vi "Delete_Overlay_2Images-2.vi"(0 "Delete \nOverlay?":bool, 1 "1st Image IN":T1, 2 "2nd Image IN":T1, 3 "error IN":errorcluster, 4 "Stored Overlay":T1) -> (5 "1st Image OUT":T1, 6 "2nd Image OUT":T1, 7 "error OUT":errorcluster)   [LabVIEW 2013]
uses:
  <vilib>/vision/Image Controls.llb/IMAQ Image.ctl
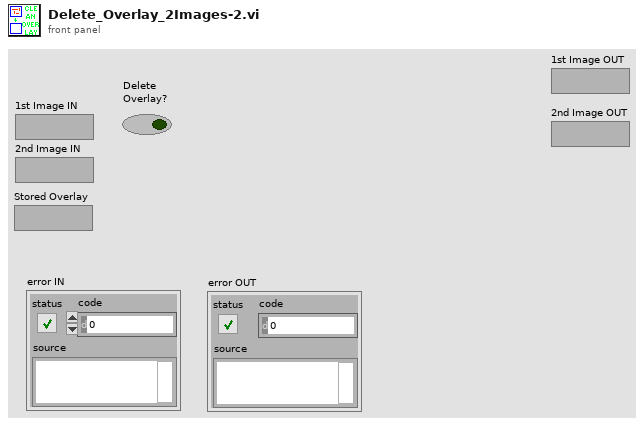
[diagram p1: front panel]
types:
  T1 = typedef "IMAQ Image.ctl" = refnum<image>
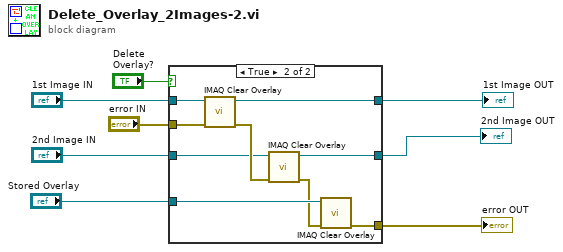
[diagram p0: block diagram]
diagram:
  n1 = case shown="True" "Delete \nOverlay?" {
    tunnel: "1st Image IN" -> [w10 w20]
    tunnel: [w10 w18] -> w6
    tunnel: "error IN" -> [w11 w19]
    tunnel: [w9 w17] -> w2
    tunnel: [w11 w12] -> w4
    tunnel: "2nd Image IN" -> [w9 w15]
    tunnel: "Stored Overlay" -> [_ w14]
    frame False {
    }
    frame True {
      n2 = call "IMAQ Clear Overlay"("error in (no error)"=w19, "Image"=w20) -> ("error out"=w16:errorcluster, "Image Out"=w18:T1)  [unwired: 8 in]
      n3 = call "IMAQ Clear Overlay"("error in (no error)"=w16, "Image"=w15) -> ("error out"=w13:errorcluster, "Image Out"=w17:T1)  [unwired: 8 in]
      n4 = call "IMAQ Clear Overlay"("error in (no error)"=w13, "Image"=w14) -> ("error out"=w12:errorcluster)  [unwired: 8 in, 1 out]
    }
  }
  "1st Image OUT" <- w6
  "error OUT" <- w4
  "2nd Image OUT" <- w2
